vi "onStart.vi"(8 "error in (no error)":errorcluster, 11 "SMO":refnum<class "SMO.lvclass">) -> (0 "error out":errorcluster, 3 "SMO out":refnum<class "SMO.lvclass">)   [LabVIEW 2013, in "SMO.lvclass"]
uses:
  SMO.lvclass
  SMO.lvclass/SMO.ctl
  Dependency/Dependency.lvclass/Dependency.ctl
  Private/ReftoDVR--SMO.vi
  Dependency/Dependency.lvclass
panel:
  # "For instructions on how to use the JKI State Machine Objects, examples and video tutorials, visit:\nhttp://jki.net/state-machine-objects/\n\nJKI State Machine Objects™\nhttp://jki.net/state-machine-objects/\nCopyright (C) 2005-2015, JKI <info@jki.net>\nALL RIGHTS RESERVED"
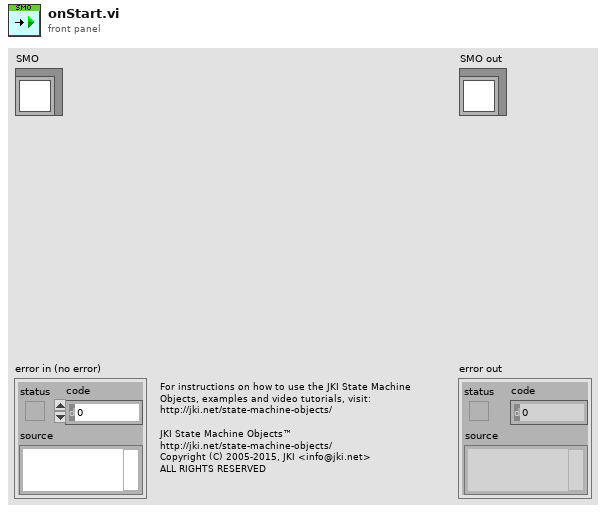
[diagram p1: front panel]
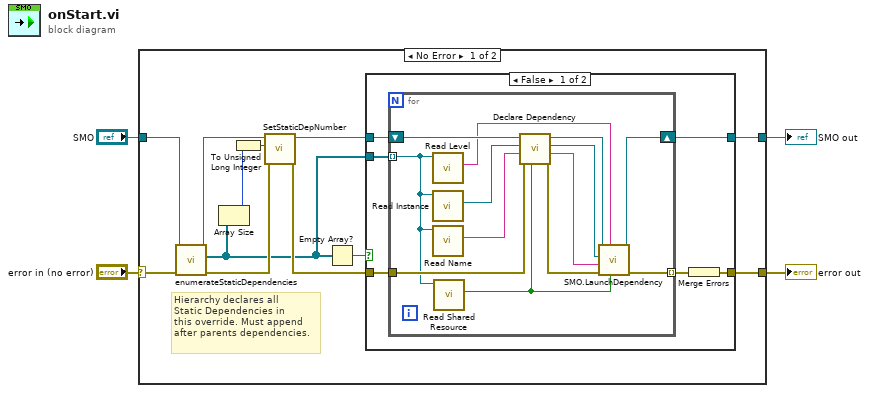
[diagram p0: block diagram]
diagram:
  n1 = case shown="No Error" "error in (no error)" {
    selector: "error in (no error)" -> [w13 w39]
    tunnel: [w15 w39] -> w3
    tunnel: [w16 w38] -> w1
    tunnel: "SMO" -> [w14 w38]
    frame No Error {
      # "Hierarchy declares all\nStatic Dependencies in\nthis override. Must append\nafter parents dependencies."
      n2 = call-dynamic "enumerateStaticDependencies.vi"("error in (no error)"=w13, "SMO"=w14) -> ("error out"=w11:errorcluster, "Static Dependencies"=w5:refnum<class "Dependency.lvclass">[], "SMO out"=w9:refnum<class "SMO.lvclass">)  [unwired: 7 in]
      n3 = Array Size(array=w5) -> (size(s)=w7:i32)
      n4 = To Unsigned Long Integer(number=w7) -> (unsigned 32bit integer=w6:u32)
      n5 = call "SetStaticDepNumber.vi"("error in (no error)"=w11, "Nb of Static Dependencies"=w6, "SMO in"=w9) -> ("error out"=w10:errorcluster, "SMO out"=w8:refnum<class "SMO.lvclass">)  [unwired: 7 in]
      n6 = Empty Array?(array=w5) -> (empty?=w12:bool)
      n7 = case shown="False" w12 {
        tunnel: w5 -> [w22 _]
        tunnel: w8 -> [w17 w37]
        tunnel: w10 -> [w20 w36]
        tunnel: [w19 w37] -> w16
        tunnel: [w18 w36] -> w15
        frame False {
          n8 = for {
            tunnel: w22 -> [w23] mode=indexing
            tunnel: w20 -> [w31]
            tunnel: [w35] -> w21 mode=indexing
            shift-right: [w34] -> w19
            shift-left: w17 -> [w33]
            n9 = call "Read Level.vi"("Dependency in"=w23) -> ("Level"=w24:string)  [unwired: 9 in, 1 out]
            n10 = call "Read Instance.vi"("Dependency in"=w23) -> ("SMO.lvclass"=w32:refnum<class "SMO.lvclass">)  [unwired: 9 in, 1 out]
            n11 = call "Read Name.vi"("Dependency in"=w23) -> ("Name"=w29:string)  [unwired: 9 in, 1 out]
            n12 = call "Read Shared Resource.vi"("Dependency in"=w23) -> ("Shared Resource"=w30:bool)  [unwired: 9 in, 1 out]
            n13 = call "Declare Dependency.vi"("Shared Resource"=w30, "error in (no error)"=w31, "Name"=w29, "Dependency"=w32, "SMO in"=w33) -> ("error out"=w25:errorcluster, "Unique Name"=w26:string, "Dependency out"=w27:refnum<class "SMO.lvclass">, "SMO out"=w28:refnum<class "SMO.lvclass">)  [unwired: 3 in]
            n14 = call "SMO.LaunchDependency.vi"("Shared Resource"=w30, "Level"=w24, "error in (no error)"=w25, "Dependency Name"=w26, "Dependency Type"=w27, "SMO in"=w28) -> ("error out"=w35:errorcluster, "SMO out"=w34:refnum<class "SMO.lvclass">)  [unwired: 2 in, 2 out]
          }
          n15 = Merge Errors(w21) -> (w18:errorcluster)
        }
        frame True {
        }
      }
    }
    frame Error {
    }
  }
  "error out" <- w3
  "SMO out" <- w1
